vi "Do.vi"(8 "error in (no error)":errorcluster, 9 "CommandQueueIn":refnum<queue>, 10 "DataNotifierIn":refnum<notifier>, 11 "CommandCopy in":refnum<class "Close.lvclass">) -> (0 "error out":errorcluster, 1 "ExitFlag":bool, 2 "DataNotifierOut":refnum<notifier>, 3 "CommandCopy out":refnum<class "Close.lvclass">)   [LabVIEW 2013, in "Close.lvclass"]
uses:
  Close.lvclass
  SystemData.lvclass/SystemData.lvclass
  RootCommand.lvclass/RootCommand.lvclass
  SystemData.lvclass/SystemData.lvclass/SystemData.ctl
  Generator.lvclass/Generator.lvclass
panel:
  # "notifier包裝SystemData物件的參考"
  # "命令物件序列參考"
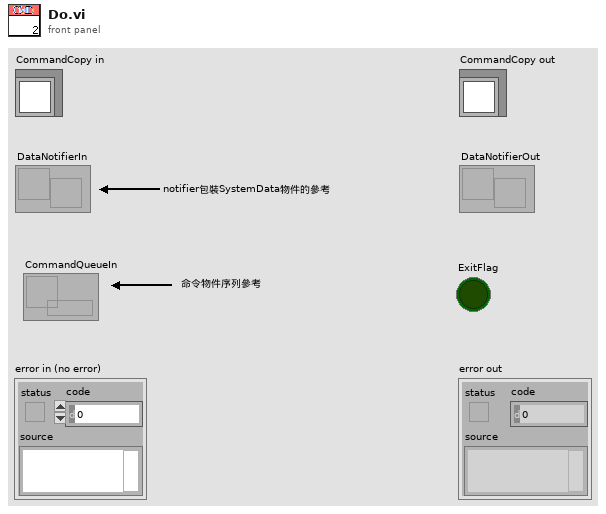
[diagram p1: front panel]
types:
  T1 = typedef "SystemData.lvclass/SystemDataTypeDefine.ctl" = cluster{"ThisVIParameter":cluster{"ThisVIPath":path, "ThisVIReference":refnum<vi>, "AllControlReference":refnum<vi>[]}, "GeneratorParameter":cluster{"Frequency":dbl, "Amplitude":dbl}, "WaveformBuffer":waveform(dbl), "SourceSelect":u16, "GeneratorClassArray":refnum<class "Generator.lvclass">[]}
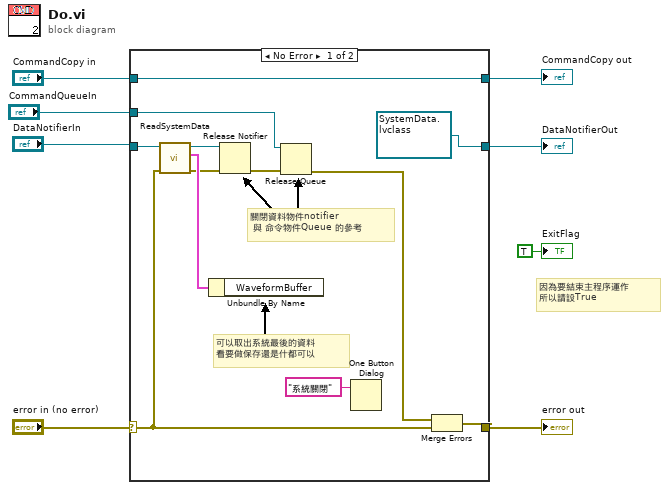
[diagram p0: block diagram]
diagram:
  # "因為要結束主程序運作\n所以請設True"
  n1 = case shown="No Error" "error in (no error)" {
    selector: "error in (no error)" -> [w16 w23]
    tunnel: [w17 w23] -> w4
    tunnel: [w20 w22] -> w3
    tunnel: "CommandCopy in" -> [w20 w22]
    tunnel: "DataNotifierIn" -> [w19 w21]
    tunnel: [refnum<notifier> refnum ("DataNotifierIn") w21] -> w2
    tunnel: "CommandQueueIn" -> [w10 _]
    frame No Error {
      # "可以取出系統最後的資料\n看要做保存還是什都可以"
      # "關閉資料物件notifier\n 與 命令物件Queue 的參考"
      n2 = call "ReadSystemData.vi"("error in (no error)"=w16, "DataNotifierIn"=w19) -> ("error out"=w15:errorcluster, "SystemData"=w18:T1, "DataNotifierIn"=w14:refnum<notifier>)  [unwired: 7 in]
      n3 = Unbundle By Name(w18) -> ()  [unwired: 1 out]
      n4 = Release Notifier(notifier=w14, error in (no error)=w15) -> (error out=w11:errorcluster)  [unwired: 1 in, 2 out]
      n5 = Release Queue(queue=w10, error in (no error)=w11) -> (error out=w9:errorcluster)  [unwired: 1 in, 2 out]
      n6 = One Button Dialog(message="系統關閉") -> ()  [unwired: 1 in, 1 out]
      n7 = Merge Errors(w9, w16) -> (w17:errorcluster)
    }
    frame Error {
    }
  }
  "error out" <- w4
  "CommandCopy out" <- w3
  "DataNotifierOut" <- w2
  "ExitFlag" <- TRUE ("ExitFlag")
